vi "Auto Hovering with Position Prediction.vi"() -> ()   [LabVIEW 2014]
uses:
  Resources/Global.vi
  <vilib>/LVH/AR Drone Toolkit/Decode Video/2.0/Decode20Video.dll
panel:
  in  "Prediction?":bool=TRUE
  out "Image":T1(plugin-control)
  out "Video Loop":errorcluster
  out "Number of Particles before":i32
  out "Number of Particles after":i32
  in  "Number of Erosion":i32=30
  out "Video refresh":u32=48
  in  "ms to wait":u32
  # "Do NOT run this VI. Instead run \"AR.Drone MAIN.vi\" and select the name of this VI in the dop-down menu at the Steup tab"
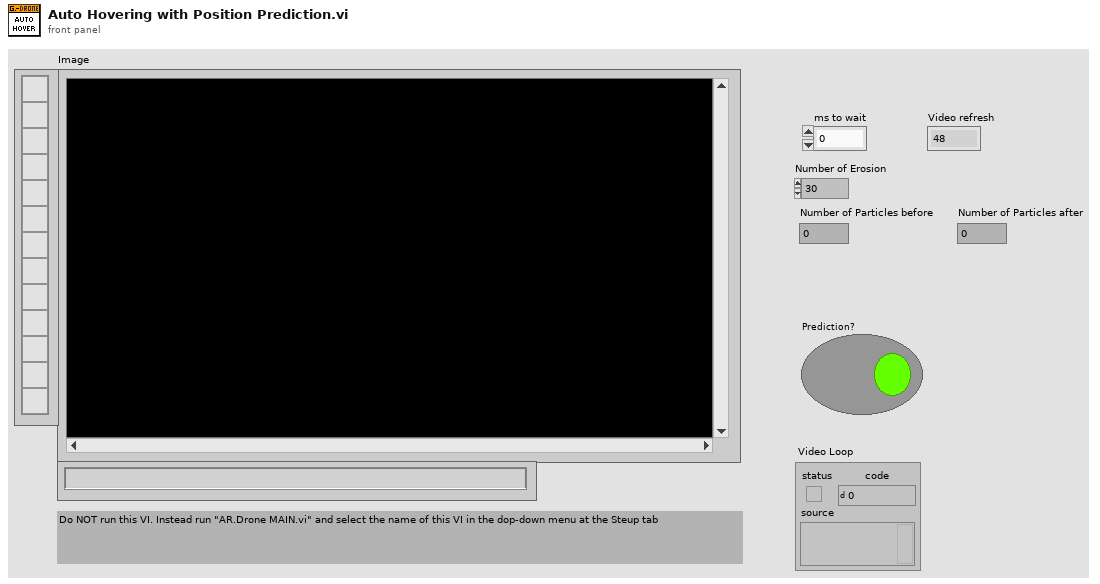
[diagram p1: front panel]
types:
  T1 = typedef "IMAQ Image.ctl" = refnum<image>
  T2 = cluster{"New Image":T1, "New Image":T1, "New Image":T1}
  T3 = cluster{"Left":dbl, "Top":dbl, "Right":dbl, "Bottom":dbl}
  T4 = cluster{"Horizontal position":dbl, "Verical position\n":dbl}
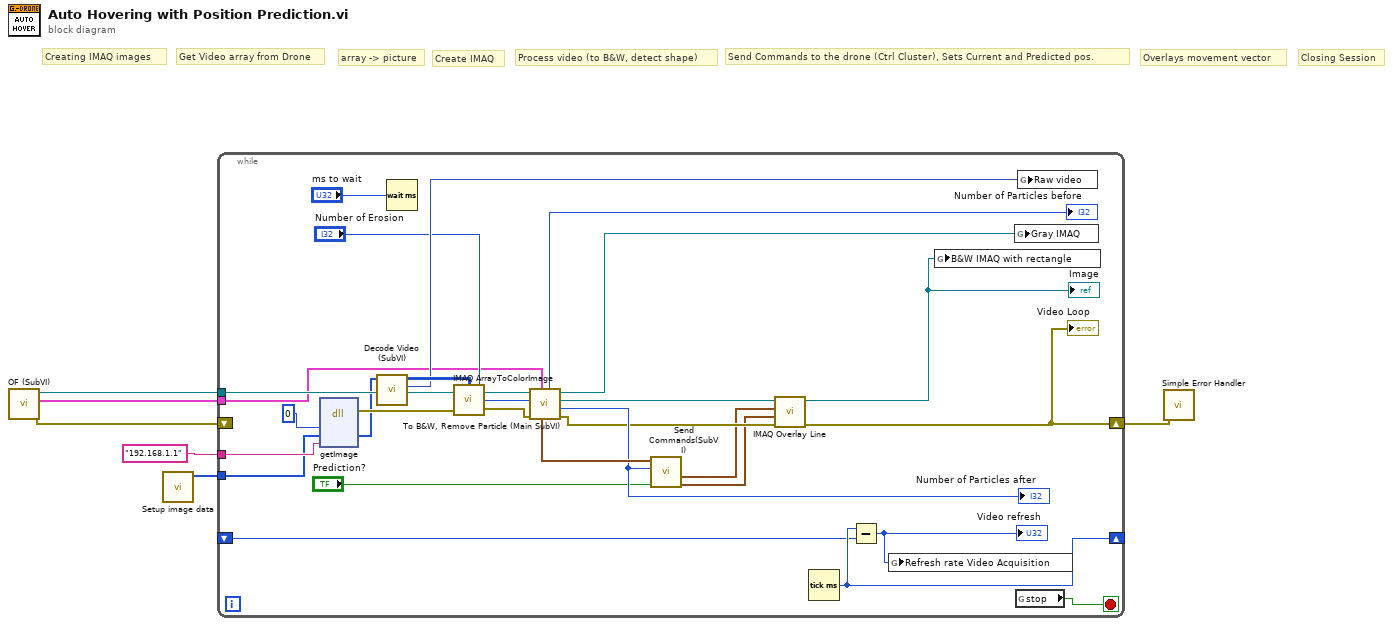
[diagram p0: block diagram]
diagram:
  # "Overlays movement vector"
  # "Send Commands to the drone (Ctrl Cluster), Sets Current and Predicted pos."
  # "Create IMAQ"
  # "Process video (to B&W, detect shape)"
  # "array -> picture"
  # "Get Video array from Drone"
  # "Closing Session"
  # "Creating IMAQ images"
  n1 = call "OF (SubVI).vi"() -> ("error out"=w4:errorcluster, "Cluster"=w5:T2, "Refnum out"=w6:T1)  [unwired: 9 in]
  n2 = call "Setup image data.vi"() -> ("Array"=w1:u8[])  [unwired: 11 in]
  n3 = while {
    shift-right: [w32] -> _
    shift-left: _ -> [w31]
    tunnel: w6 -> [w23]
    tunnel: w5 -> [w22]
    shift-right: [w14] -> w3
    shift-left: w4 -> [_]
    tunnel: "192.168.1.1" ("IP Address") -> [w9]
    tunnel: w1 -> [w8]
    stop <- w24 stop-if-true
    n4 = dll-call lib="C:/Program Files (x86)/National Instruments/LabVIEW 2014/vi.lib/LVH/AR Drone Toolkit/Decode Video/2.0/Decode20Video.dll" fn="getImage"("Index"=0, "ImgData"=w8, "IP Address"=w9) -> (error out=w12:errorcluster, "ImgData"=w11:u8[])  [unwired: 6 in, 1 out]
    n5 = call "Decode Video (SubVI).vi"("ImgData"=w11) -> ("new picture"=w30:picture, "Array"=w33:u32[][])  [unwired: 9 in]
    n6 = Wait (ms)(milliseconds to wait="ms to wait") -> ()  [unwired: 1 out]
    n7 = call "IMAQ ArrayToColorImage"("Image Pixels (U32)"=w33, "Image"=w23, "error in (no error)"=w12) -> ("Image Out"=w29:T1, "error out"=w19:errorcluster)  [unwired: 2 in]
    n8 = call "To B&W, Remove Particle (Main SubVI).vi"("Image Reference Sources"=w22, "error in (no error)"=w19, "Number of Erosion"="Number of Erosion", "Refnum in"=w29) -> ("error out"=w17:errorcluster, "Number of Particles after"=w25:i32, "Image Out"=w18:T1, "Current Grayscale"=w21:T1, "Number of Particles before"=→"Number of Particles before":i32, "Cluster"=w27:T3)  [unwired: 1 in, 1 out]
    "Number of Particles after" <- w25
    n9 = call "Send Commands(SubVI).vi"("Prediction?"="Prediction?", "Number of Particles after"=w25, "Cluster"=w27) -> ("Predicted Position"=w16:T4, "Current position"=w15:T4)  [unwired: 7 in]
    n10 = call "IMAQ Overlay Line"("error in (no error)"=w17, "End Point"=w16, "Start Point"=w15, "Image"=w18) -> ("error out"=w14:errorcluster, "Image Out"=w13:T1)  [unwired: 6 in]
    "Video Loop" <- w14
    "Image" <- w13
    n11 = Tick Count (ms)() -> (millisecond timer value=w32:u32)
    n12 = Subtract(x=w32, y=w31) -> (x-y=w7:u32)
    "Video refresh" <- w7
    n13 = global write "Global.vi" "Refresh rate Video Acquisition"(w7) -> ()
    n14 = global write "Global.vi" "B&W IMAQ with rectangle"(w13) -> ()
    n15 = global write "Global.vi" "Gray IMAQ"(w21) -> ()
    n16 = global read "Global.vi" "stop"() -> (w24:bool)
    n17 = global write "Global.vi" "Raw video"(w30) -> ()
  }
  n18 = call <vilib>:"Simple Error Handler.vi"("error in (no error)"=w3) -> ()  [unwired: 4 in, 5 out]
